vi "Write Associated GUI Class Path.vi"(8 "error in (no error)":errorcluster, 10 "Associated GUI Class Path":path, 11 "CS++BaseActor in":refnum<class "CS++BaseActor.lvclass">) -> (0 "error out":errorcluster, 3 "CS++BaseActor out":refnum<class "CS++BaseActor.lvclass">)   [LabVIEW 2014, in "CS++BaseActor.lvlib" / "CS++BaseActor.lvclass"]
doc: "Write LVClassPath of the GUI correponding to the device."
uses:
  CS++BaseActor.lvclass
  CS++BaseActor.lvclass/CS++BaseActor.ctl
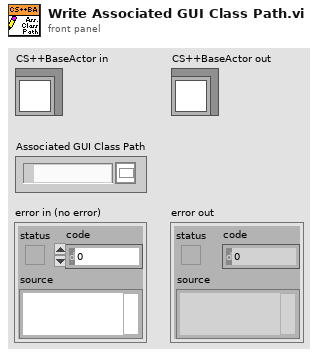
[diagram p1: front panel]
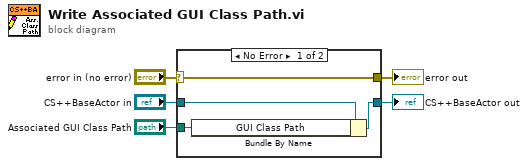
[diagram p0: block diagram]
diagram:
  n1 = case shown="No Error" "error in (no error)" {
    selector: "error in (no error)" -> [w9 w10]
    tunnel: [w9 w10] -> w4
    tunnel: [w7 w11] -> w2
    tunnel: "CS++BaseActor in" -> [w8 w11]
    tunnel: "Associated GUI Class Path" -> [w6 _]
    frame No Error {
      n2 = Bundle By Name(cluster=w8, "GUI Class Path"=w6) -> (w7:refnum<class "CS++BaseActor.lvclass">)
    }
    frame Error {
    }
  }
  "error out" <- w4
  "CS++BaseActor out" <- w2
